vi "Linearly Spaced Array 2012 NIVerified.vi"(8 "error in (no error)":errorcluster, 9 "Number of Samples":i32, 10 "End":dbl, 11 "Start":dbl) -> (0 "error out":errorcluster, 3 "Array":dbl[](array[numeric]))   [LabVIEW 2024, in "Sweep.lvlib"]
doc: "This subVI will create an evenly spaced array of elements equal to the Number of Samples between the Minimum and Maximum"
uses:
  Sweep.lvlib
panel:
  # "Overview: Generate array with equally spaced array elements.\nRequirements: LabVIEW Full Development System\nInstructions:\n1- Enter the minimum value (start value)\n2- Enter the maximum value (end value)\n3- Enter the number of samples (number of elements)\n4- Run the VI"
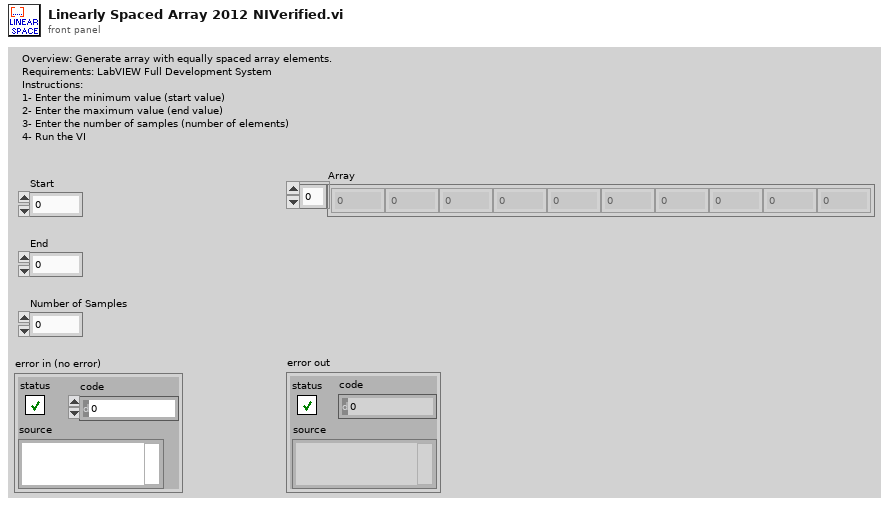
[diagram p1: front panel]
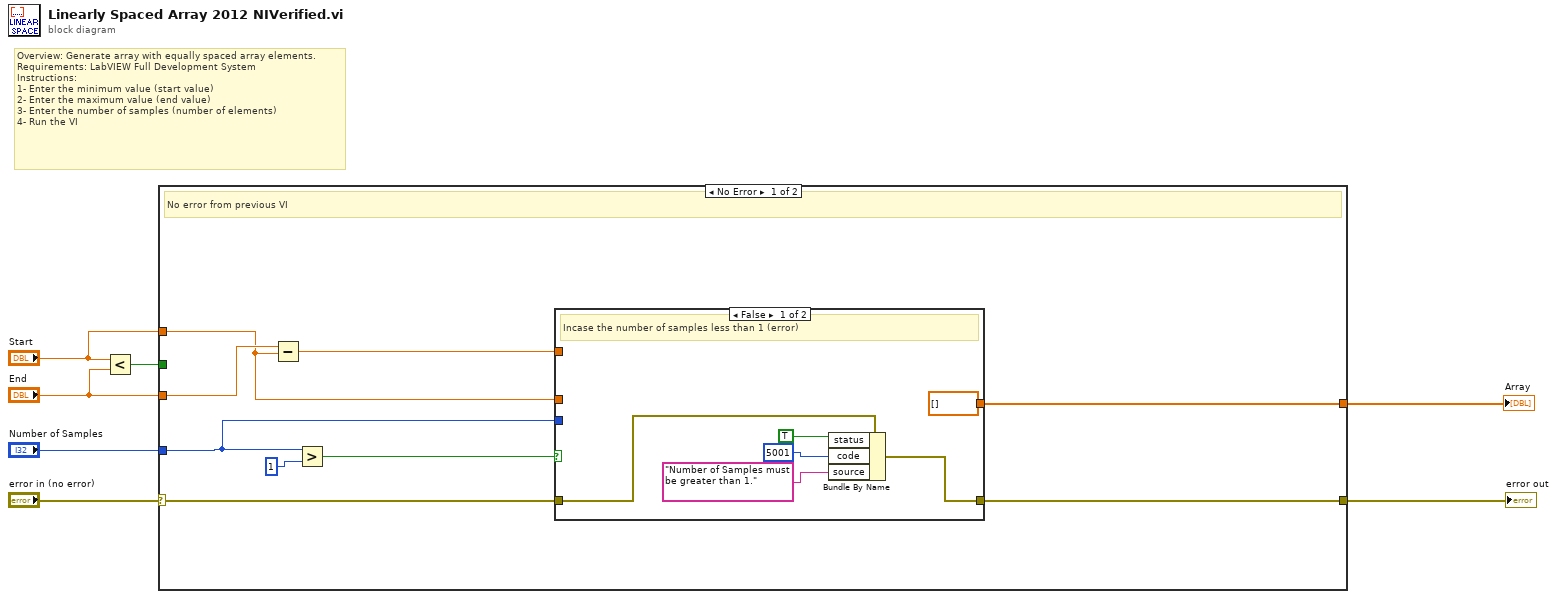
[diagram p0: block diagram]
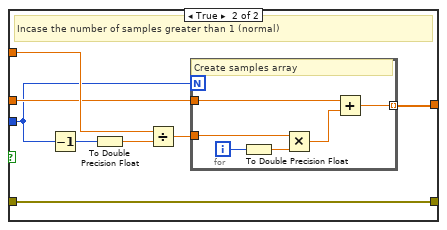
[diagram p2: hidden frame]
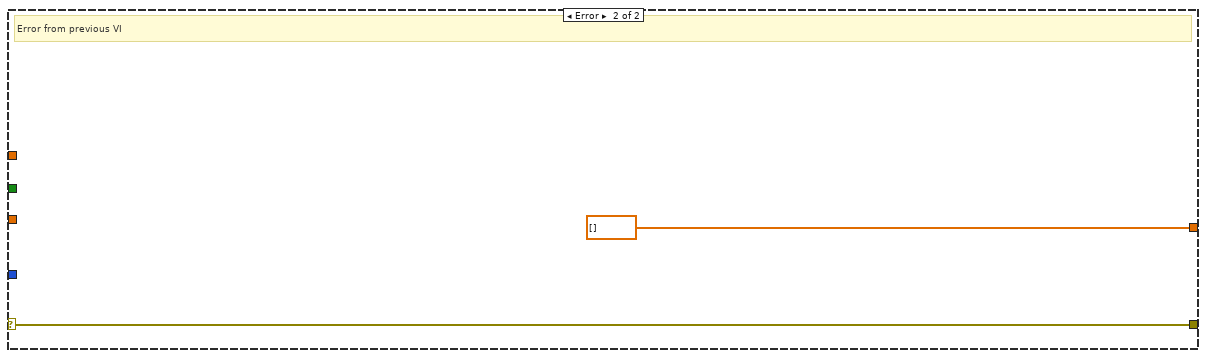
[diagram p3: hidden frame]
diagram:
  # "Overview: Generate array with equally spaced array elements.\nRequirements: LabVIEW Full Development System\nInstructions:\n1- Enter the minimum value (start value)\n2- Enter the maximum value (end value)\n3- Enter the number of samples (number of elements)\n4- Run the VI"
  n1 = Less?(x="Start", y="End") -> (x < y?=w7:bool)
  n2 = case shown="No Error" "error in (no error)" {
    selector: "error in (no error)" -> [w12 w37]
    tunnel: w7 -> [_ _]
    tunnel: "End" -> [w16 _]
    tunnel: "Start" -> [w15 _]
    tunnel: [w14 w37] -> w1
    tunnel: "Number of Samples" -> [w13 _]
    tunnel: [w11 dbl[] []] -> w5
    frame No Error {
      # "No error from previous VI"
      n3 = Subtract(x=w16, y=w15) -> (x-y=w10:dbl)
      n4 = Greater?(x=w13, y=1) -> (0:w8:bool)
      n5 = case shown="False" w8 {
        tunnel: w10 -> [_ w30]
        tunnel: w12 -> [w22 w29]
        tunnel: [w21 w29] -> w14
        tunnel: w13 -> [_ w24]
        tunnel: w15 -> [_ w26]
        tunnel: [dbl[] [] w25] -> w11
        frame False {
          # "Incase the number of samples less than 1 (error)"
          n6 = Bundle By Name(cluster=w22, "status"=TRUE, "code"=5001, "source"="Number of Samples must be greater than 1.") -> (w21:errorcluster)
        }
        frame True {
          # "Incase the number of samples greater than 1 (normal)"
          n7 = Decrement(x=w24) -> (x-1=w28:i32)
          n8 = To Double Precision Float(number=w28) -> (double precision float=w23:dbl)
          n9 = Divide(x=w30, y=w23) -> (x/y=w27:dbl)
          n10 = for {
            N: w24 -> [_]
            tunnel: w26 -> [w32]
            tunnel: w27 -> [w35]
            tunnel: [w34] -> w25 mode=indexing
            i -> [w36]
            # "Create samples array"
            n11 = To Double Precision Float(number=w36) -> (double precision float=w33:dbl)
            n12 = Multiply(x=w35, y=w33) -> (x*y=w31:dbl)
            n13 = Add(x=w32, y=w31) -> (x+y=w34:dbl)
          }
        }
      }
    }
    frame Error {
      # "Error from previous VI"
    }
  }
  "error out" <- w1
  "Array" <- w5
